vi "GetFPObjTypes.vi"(8 "error in (no error)":errorcluster, 11 "VI in":refnum<vi>) -> (0 "error out":errorcluster, 2 "Object Types":string[](array[string]), 3 "reference out":refnum<vi>)   [LabVIEW 2014]
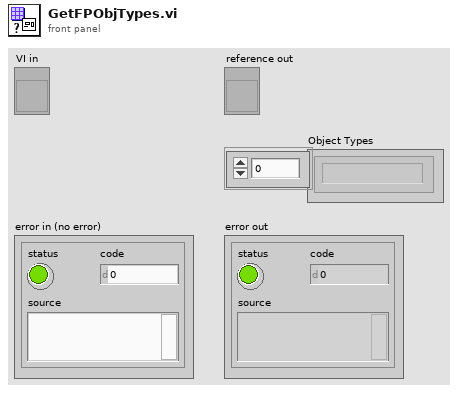
[diagram p1: front panel]
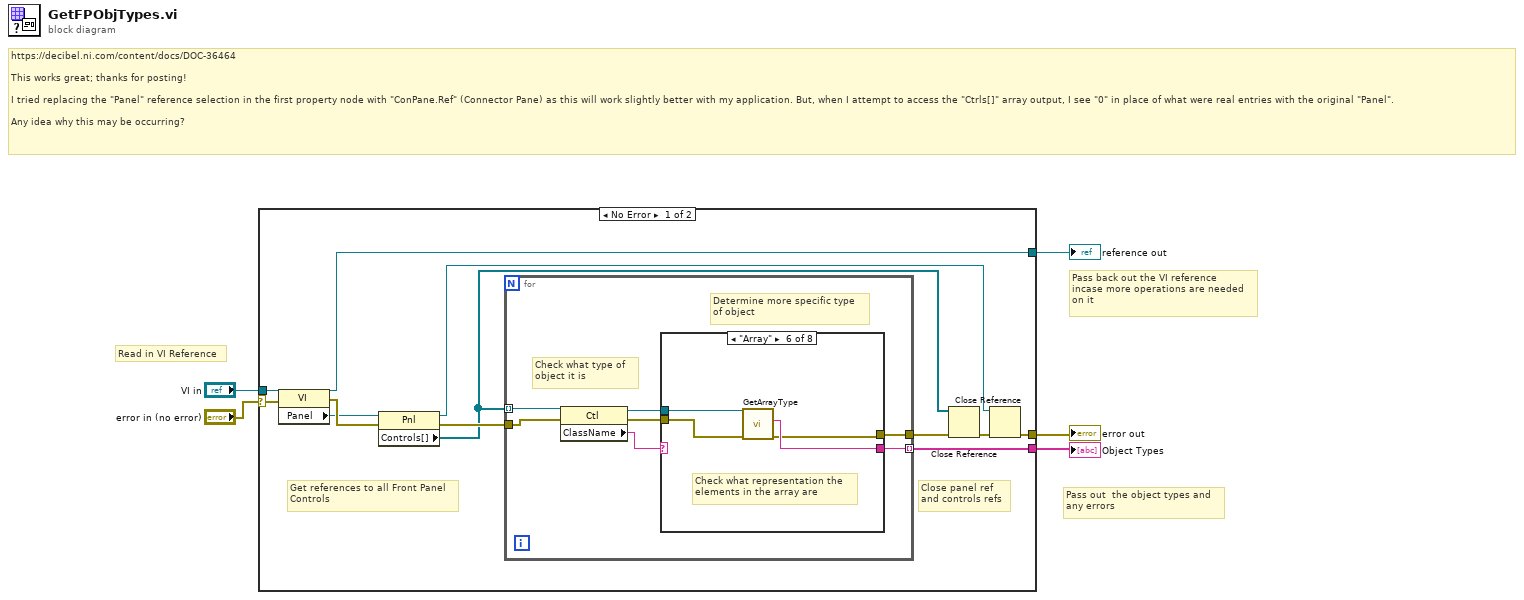
[diagram p0: block diagram]
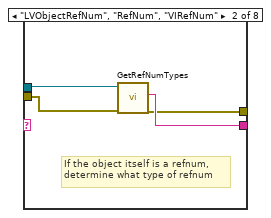
[diagram p3: hidden frame]
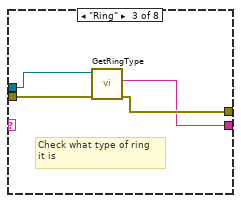
[diagram p4: hidden frame]
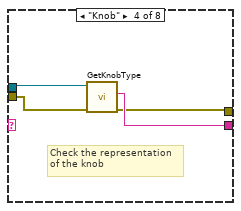
[diagram p5: hidden frame]
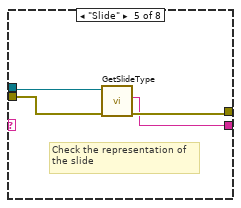
[diagram p6: hidden frame]
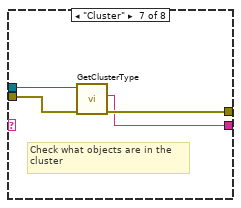
[diagram p7: hidden frame]
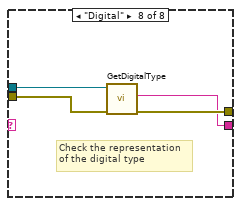
[diagram p8: hidden frame]
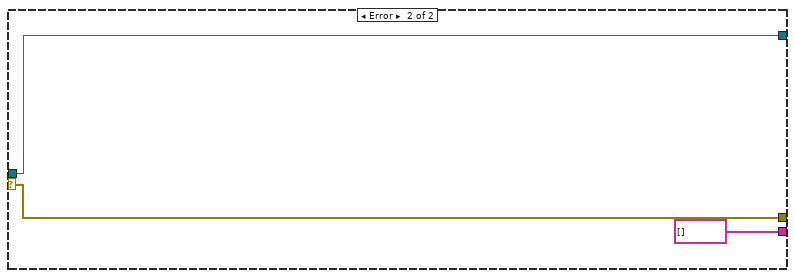
[diagram p9: hidden frame]
diagram:
  # "https://decibel.ni.com/content/docs/DOC-36464\n\nThis works great; thanks for posting!\n\nI tried replacing the \"Panel\" reference selection in the first property node with \"ConPane.Ref\" (Connector Pane) as this will work slightly better with my application. But, when I attempt to access the \"Ctrls[]\" array output, I see \"0\" in place of what were real entries with the original \"Panel\".\n\nAny idea why this may be occurring?"
  # "Pass back out the VI reference\nincase more operations are needed\non it"
  # "Pass out  the object types and\nany errors"
  # "Read in VI Reference"
  n1 = case shown="No Error" "error in (no error)" {
    selector: "error in (no error)" -> [w10 w57]
    tunnel: [w7 w57] -> w5
    tunnel: [w15 string[] []] -> w4
    tunnel: "VI in" -> [w14 w55]
    tunnel: [w11 w55] -> w2
    frame No Error {
      # "Close panel ref\nand controls refs"
      # "Get references to all Front Panel\nControls"
      n2 = property class="VI"(reference=w14, error in=w10) -> (reference out=w11:refnum<vi>, error out=w13:errorcluster, "Panel"=w12:refnum<vi>)
      n3 = property class="Pnl"(reference=w12, error in=w13) -> (reference out=w6:refnum<vi>, error out=w16:errorcluster, "Controls[]"=w8:refnum<vi>[])
      n4 = for {
        tunnel: w8 -> [w24] mode=indexing
        tunnel: [w20] -> w15 mode=indexing
        tunnel: w16 -> [w19]
        tunnel: [w18] -> w17
        # "Determine more specific type\nof object"
        # "Check what type of\nobject it is"
        n5 = property class="Ctl"(reference=w24, error in=w19) -> (reference out=w22:refnum<vi>, error out=w21:errorcluster, "ClassName"=w23:string)
        n6 = case shown="\"Array\"" w23 {
          selector: w23 -> [w25 _ _ _ _ _ _ _]
          tunnel: w22 -> [_ w29 w33 w35 w42 w46 w50 w53]
          tunnel: w21 -> [w26 w30 w34 w38 w41 w45 w49 w54]
          tunnel: [w25 w28 w31 w37 w39 w44 w47 w51] -> w20
          tunnel: [w26 w27 w32 w36 w40 w43 w48 w52] -> w18
          frame Default {
            # "If other object, just pass through\nclass name"
          }
          frame "LVObjectRefNum", "RefNum", "VIRefNum" {
            # "If the object itself is a refnum,\ndetermine what type of refnum"
            n7 = call "GetRefNumTypes.vi"("error in (no error)"=w30, "Control in"=w29) -> ("error out"=w27:errorcluster, "RefNumType"=w28:string)  [unwired: 7 in, 1 out]
          }
          frame "Ring" {
            # "Check what type of ring\nit is"
            n8 = call "GetRingType.vi"("error in (no error)"=w34, "Control Ref In"=w33) -> ("error out"=w32:errorcluster, "Ring Type"=w31:string)  [unwired: 7 in, 1 out]
          }
          frame "Knob" {
            # "Check the representation\nof the knob"
            n9 = call "GetKnobType.vi"("error in (no error)"=w38, "reference in"=w35) -> ("error out"=w36:errorcluster, "Knob Type"=w37:string)  [unwired: 7 in, 1 out]
          }
          frame "Slide" {
            # "Check the representation of\nthe slide"
            n10 = call "GetSlideType.vi"("error in (no error)"=w41, "Control in"=w42) -> ("error out"=w40:errorcluster, "Knob Type"=w39:string)  [unwired: 7 in, 1 out]
          }
          frame "Array" {
            # "Check what representation the\nelements in the array are"
            n11 = call "GetArrayType.vi"("error in (no error)"=w45, "Control in"=w46) -> ("error out"=w43:errorcluster, "Type"=w44:string)  [unwired: 7 in, 1 out]
          }
          frame "Cluster" {
            # "Check what objects are in the \ncluster"
            n12 = call "GetClusterType.vi"("error in"=w49, "Control in"=w50) -> ("error out"=w48:errorcluster, "Cluster Type"=w47:string)  [unwired: 7 in, 1 out]
          }
          frame "Digital" {
            # "Check the representation\nof the digital type"
            n13 = call "GetDigitalType.vi"("error in (no error)"=w54, "Control in"=w53) -> ("error out"=w52:errorcluster, "String"=w51:string)  [unwired: 7 in, 1 out]
          }
        }
      }
      n14 = Close Reference(reference=w8, error in (no error)=w17) -> (error out=w9:errorcluster)
      n15 = Close Reference(reference=w6, error in (no error)=w9) -> (error out=w7:errorcluster)
    }
    frame Error {
    }
  }
  "error out" <- w5
  "Object Types" <- w4
  "reference out" <- w2
